vi "Smart Open.vi"(7 "Allow multiple opens?":bool=TRUE, 8 "error in (no error)":errorcluster, 10 "Channel Names":tag[](array[tag])) -> (0 "error out":errorcluster, 3 "AO (N Samples) Ref Out":T1)   [LabVIEW 2021, in "AO Block.lvlib"]
doc: "Opens a reference to analog output block write channel (ConnectorA/AO0). You must open a reference before you write values to the analog output block write channel."
uses:
  <vilib>/myRIO/Instrument Drivers/Onboard IO/AO Block/AO Block.lvlib
  <vilib>/myRIO/Common/Instrument Driver Framework/Utilities/typedefs/Hardware Version Enum.ctl
  <vilib>/myRIO/Common/Instrument Driver Framework/Utilities/typedefs/Generic FPGA Reference.ctl
  <vilib>/myRIO/Common/Instrument Driver Framework/Utilities/typedefs/myRIO v1.0 Reference.ctl
  <vilib>/myRIO/Common/Instrument Driver Framework/Utilities/typedefs/myRIO Generic Hardware Reference.ctl
  <vilib>/myRIO/Common/Instrument Driver Framework/myRIO v1.0/AO Block/typedefs/AO Block Channels Enum.ctl
  <vilib>/myRIO/Common/Instrument Driver Framework/myRIO v1.0/AO Block/typedefs/AO Block Channels List.ctl
  <vilib>/myRIO/Instrument Drivers/Onboard IO/AO Block/typedefs/AO Block Reference.ctl
  <vilib>/myRIO/Common/Instrument Driver Framework/Utilities/typedefs/Analog Scaling Constants.ctl
  <vilib>/myRIO/Instrument Drivers/Onboard IO/AO Block/vis/myRIO AO N Samples Open.xnode
  <vilib>/myRIO/Common/Instrument Driver Framework/myRIO v1.0/AO Block/vis/myRIO v1.1 Open Throughput AO (N Samples).vi
  <vilib>/userdefined/High Color/nirio_resource_hc.ctl
  <vilib>/myRIO/Instrument Drivers/Utilities/Utilities.lvlib
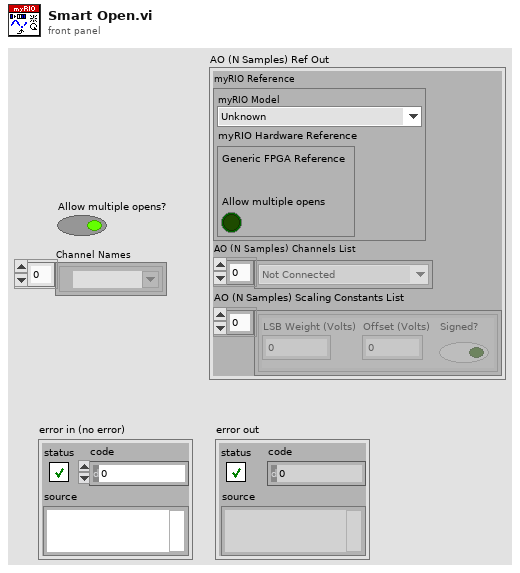
[diagram p1: front panel]
types:
  T1 = typedef "AO Block.lvlib/AO Block Reference.ctl" = cluster{"myRIO Reference":T2, "AO (N Samples) Channels List":T6, "AO (N Samples) Scaling Constants List":T8[]}
  T2 = typedef "myRIO Generic Hardware Reference.ctl" = cluster{"myRIO Model":T3, "myRIO Hardware Reference":T4}
  T3 = typedef "Hardware Version Enum.ctl" = enum16{"Unknown", "myRIO-1900", "myRIO-1950", "roboRIO", "NI ELVIS RIO CM", "ELVIS III"}
  T4 = typedef "myRIO v1.0 Reference.ctl" = cluster{"Generic FPGA Reference":T5, "Allow multiple opens":bool}
  T5 = typedef "Generic FPGA Reference.ctl" = refnum<k20>
  T6 = typedef "AO Block Channels List.ctl" = T7[]
  T7 = typedef "AO Block Channels Enum.ctl" = enum16{"Not Connected", "A/AO0 (N Samples)", "A/AO1 (N Samples)", "B/AO0 (N Samples)", "B/AO1 (N Samples)"}
  T8 = typedef "Analog Scaling Constants.ctl" = cluster{"LSB Weight (Volts)":dbl, "Offset (Volts)":dbl, "Signed?":bool}
  T9 = typedef "nirio_resource_hc.ctl" = tag
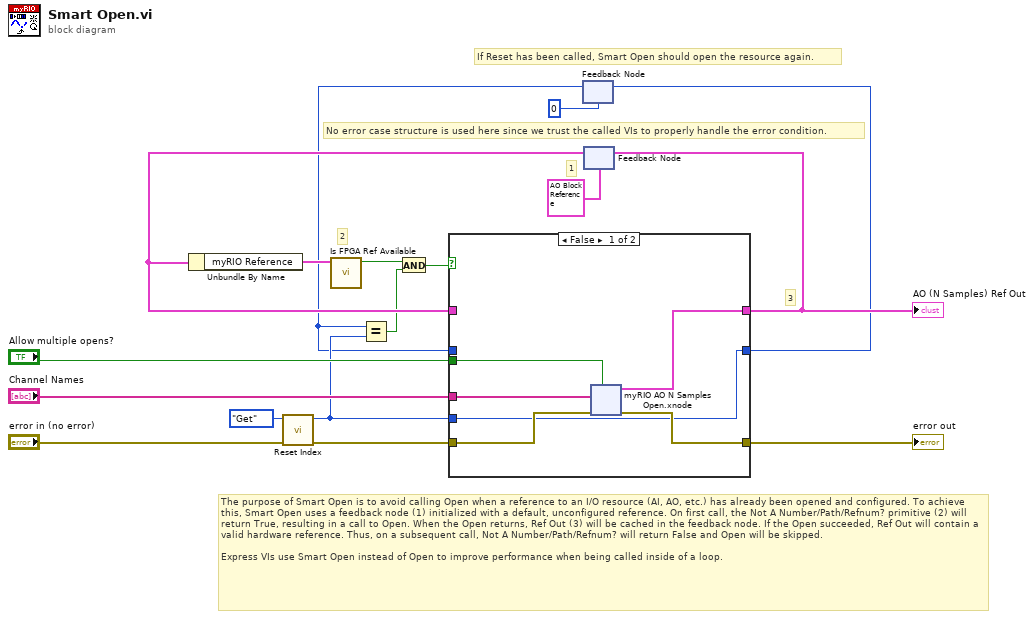
[diagram p0: block diagram]
diagram:
  # "If Reset has been called, Smart Open should open the resource again."
  # "No error case structure is used here since we trust the called VIs to properly handle the error condition."
  # "3"
  # "1"
  # "2"
  # "The purpose of Smart Open is to avoid calling Open when a reference to an I/O resource (AI, AO, etc.) has already been opened and configured. To achieve this, Smart Open uses a feedback node (1) initialized with a default, unconfigured reference. On first call, the Not A Number/Path/Refnum? primitive (2) will return True, resulting in a call to Open. When the Open returns, Ref Out (3) will be cached in the feedback node. If the Open succeeded, Ref Out will contain a valid hardware reference. Thus, on a subsequent call, Not A Number/Path/Refnum? will return False and Open will be skipped.\n\t\nExpress VIs use Smart Open instead of Open to improve performance when being called inside of a loop."
  n1 = call <vilib>:"Reset Index.vi"("error in (no error)"="error in (no error)", "Action"=enum16{"Get", "Set"}."Get") -> ("error out"=w9:errorcluster, "Ref Count"=w6:u8)  [unwired: 8 in]
  n2 = feedback #1(u8 0 ("Ref Count")) -> (w5:u8)
  n3 = Equal?(x=w5, y=w6) -> (x = y?=w3:bool)
  n4 = feedback #2(T1 {"myRIO Reference"={"myRIO Model"=enum."Unknown", "myRIO Hardware Reference"={"Generic FPGA Reference"=refnum, "Allow multiple opens"=FALSE}}, "AO (N Samples) Channels List"=[], "AO (N Samples) Scaling Constants List"=[]} ("AI (N Samples) Read Ref Out")) -> (w17:T1)
  n5 = Unbundle By Name(w17) -> ("myRIO Reference"=w11:T2)
  n6 = call <vilib>:"Is FPGA Ref Available.vi"("myRIO Reference"=w11) -> ("Is Available?"=w4:bool)  [unwired: 10 in]
  n7 = And(x=w4, y=w3) -> (x .and. y?=w2:bool)
  n8 = case shown="False" w2 {
    tunnel: w9 -> [w23 w43]
    tunnel: [w22 w44] -> w14
    tunnel: [w21 w43] -> w16
    tunnel: w17 -> [_ w44]
    tunnel: "Channel Names" -> [w20 _]
    tunnel: "Allow multiple opens?" -> [w19 _]
    tunnel: [w18 w42] -> w8
    tunnel: w5 -> [_ w42]
    tunnel: w6 -> [w18 _]
    frame False {
      n9 = xnode "myRIO AO N Samples Open.xnode"("error in (no error)"=w23, "Allow multiple opens?"=w19, "Channel Names"=w20) -> ("error out"=w21:errorcluster, "AO (N Samples) Ref Out"=w22:T1)
    }
    frame True {
    }
  }
  "AO (N Samples) Ref Out" <- w14
  "error out" <- w16
  n10 = feedback-in #1(w8) -> ()
  n11 = feedback-in #2(w14) -> ()
